vi "SENS_IF_FILT_STAGE_FREQ.vi"(0 "VISA IN":refnum<visa-resource-name>, 1 "Stage 1 Frq.":i32, 5 "error in":errorcluster, 7 "Channel":i32) -> (14 "VISA Out":refnum<visa-resource-name>, 19 "error out":errorcluster)   [LabVIEW 2018, in "PNA-X.lvlib"]
doc: "SENSe<cnum>:IF:FILTer:STAGE1:FREQuency <value> \n(Read-Write) Sets and returns the Numerically Controlled Oscillator (NCO) frequency. This command \nis only used when SENSe:IF:FILTer:AUTO is set to False (Manual). \nCritical Note \nParameters \n<cnum> Existing channel number. If unspecified, <cnum> is set to 1. \n<value> Stage 1 Frequency. Min value= 0 Hz, Max value= 15 MHz. Or \nprogrammatically use the Max and Min queries to determine the range of \nsettable values. \nExamples SENS:IF:FILT:STAGe1:FREQ 9e6 \nsense2:if:filter:stage1:frequency 9.2e6 \nQuery Syntax SENSe<cnum>:IF:FILTer:STAGE1:FREQuency? \n'returns the current parameter value"
uses:
  PNA-X.lvlib
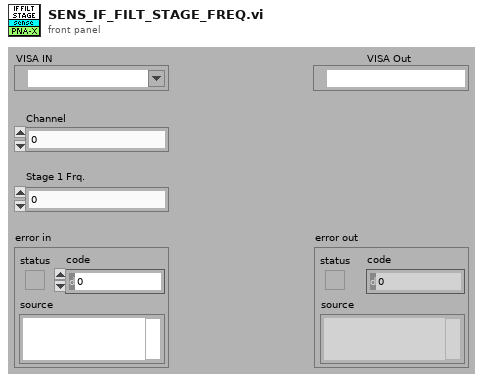
[diagram p1: front panel]
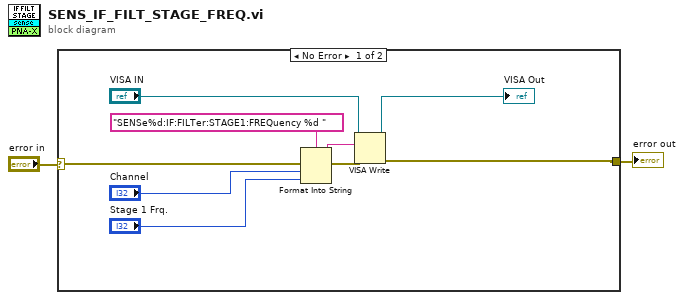
[diagram p0: block diagram]
diagram:
  n1 = case shown="No Error" "error in" {
    selector: "error in" -> [w11 w12]
    tunnel: [w6 w12] -> w1
    frame No Error {
      n2 = Format Into String(format string="SENSe%d:IF:FILTer:STAGE1:FREQuency %d " ("Cmdline"), error in=w11, "Channel", "Stage 1 Frq.") -> (resulting string=w9:string, error out=w10:errorcluster)  [unwired: 1 in]
      n3 = VISA Write(VISA resource name="VISA IN", write buffer=w9, error in (no error)=w10) -> (VISA resource name out=→"VISA Out":refnum<visa-resource-name>, error out=w6:errorcluster)  [unwired: 1 out]
    }
    frame Error {
    }
  }
  "error out" <- w1
